vi "CameraAttributeSearch.vi"() -> ()   [LabVIEW 2020]
uses:
  <vilib>/userDefined/High Color/IMAQdx.ctl
  <vilib>/vision/driver/IMAQdx.llb/IMAQdx Attribute Type.ctl
  <vilib>/vision/driver/NI_Vision_Acquisition_Software.lvlib
panel:
  out "Ready":bool=TRUE
  out "Array":T2(array[cluster])
  in  "Attribute search":string
  in  "stop":bool
  in  "Session In":T3
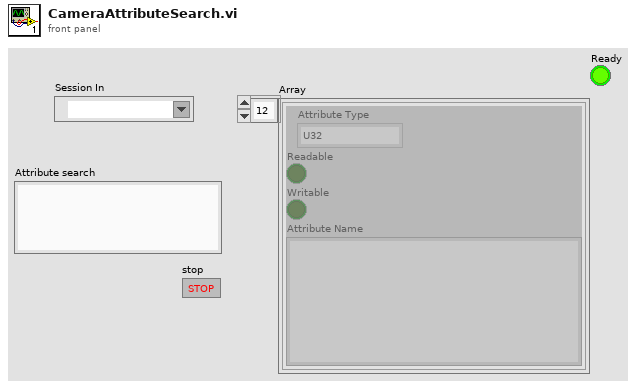
[diagram p1: front panel]
types:
  T1 = typedef "NI_Vision_Acquisition_Software.lvlib/IMAQdx Attribute Type.ctl" = enum32{"U32", "I64", "DBL", "String", "Enum", "Bool", "Command"}
  T2 = cluster{"Attribute Type":T1, "Readable":bool, "Writable":bool, "Attribute Name":string}[]
  T3 = typedef "IMAQdx.ctl" = refnum<k21>
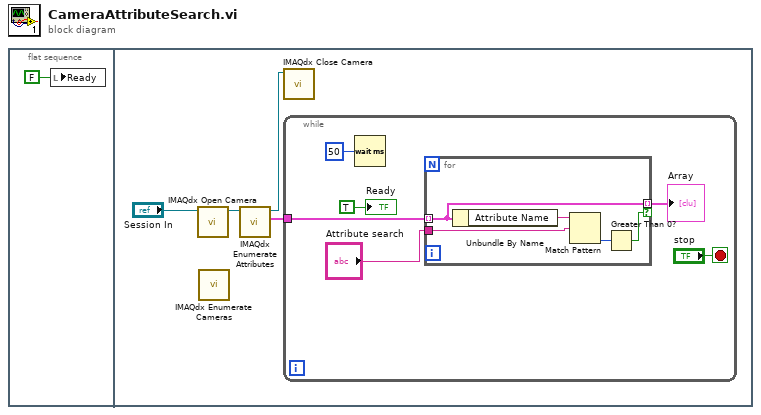
[diagram p0: block diagram]
diagram:
  n1 = flat-sequence {
    frame #0 {
      n2 = local write "Ready"(FALSE) -> ()
    }
    frame #1 {
      n3 = call <vilib>:"IMAQdx Open Camera.vi"("Session In"="Session In") -> ("Session Out"=w5:T3)  [unwired: 9 in, 1 out]
      n4 = call <vilib>:"IMAQdx Enumerate Cameras.vi"() -> ()  [unwired: 10 in, 2 out]
      n5 = call <vilib>:"IMAQdx Enumerate Attributes.vi"("Session In"=w5) -> ("Attribute Information Array"=w3:T2, "Session Out"=w4:T3)  [unwired: 8 in, 1 out]
      n6 = call <vilib>:"IMAQdx Close Camera.vi"("Session In"=w4) -> ()  [unwired: 10 in, 1 out]
      n7 = while {
        tunnel: w3 -> [w9]
        stop <- "stop" stop-if-true
        n8 = Wait (ms)(milliseconds to wait=u32 50) -> ()  [unwired: 1 out]
        n9 = for {
          tunnel: w9 -> [w12] mode=indexing
          tunnel: "Attribute search" -> [w15]
          tunnel: [w12] -> w7 mode=indexing if=w13
          n10 = Unbundle By Name(w12) -> ("Attribute Name"=w16:string)
          n11 = Match Pattern(string=w16, regular expression=w15) -> (offset past match=w14:i32)  [unwired: 1 in, 3 out]
          n12 = Greater Than 0?(x=w14) -> (x > 0?=w13:bool)
        }
        "Array" <- w7
        "Ready" <- TRUE
      }
    }
  }
